vi "Update RPC Client Methods.vi"(7 "RPC Method Parameters":T1[](array[typedef]), 8 "error in (no error)":errorcluster, 11 "Server class in":refnum<vi>) -> (0 "error out":errorcluster, 3 "Server class out":refnum<vi>)   [LabVIEW 2019, in "gRPC Template Creation Utility.lvlib"]
uses:
  gRPC Template Creation Utility.lvlib
  TypeDefs/RPC Method Parameters.ctl
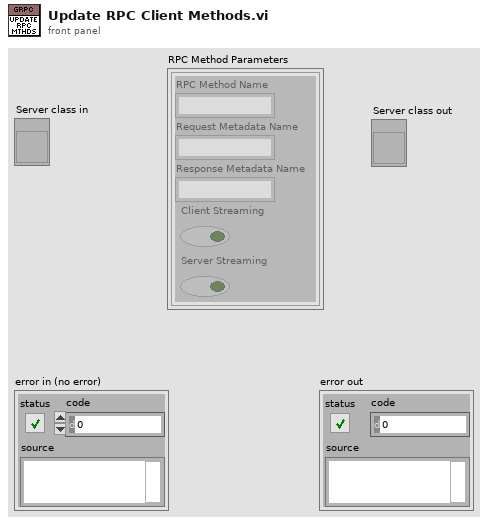
[diagram p1: front panel]
types:
  T1 = typedef "gRPC Template Creation Utility.lvlib/RPC Method Parameters.ctl" = cluster{"RPC Method Name":string, "Request Metadata Name":string, "Response Metadata Name":string, "Client Streaming":bool, "Server Streaming":bool}
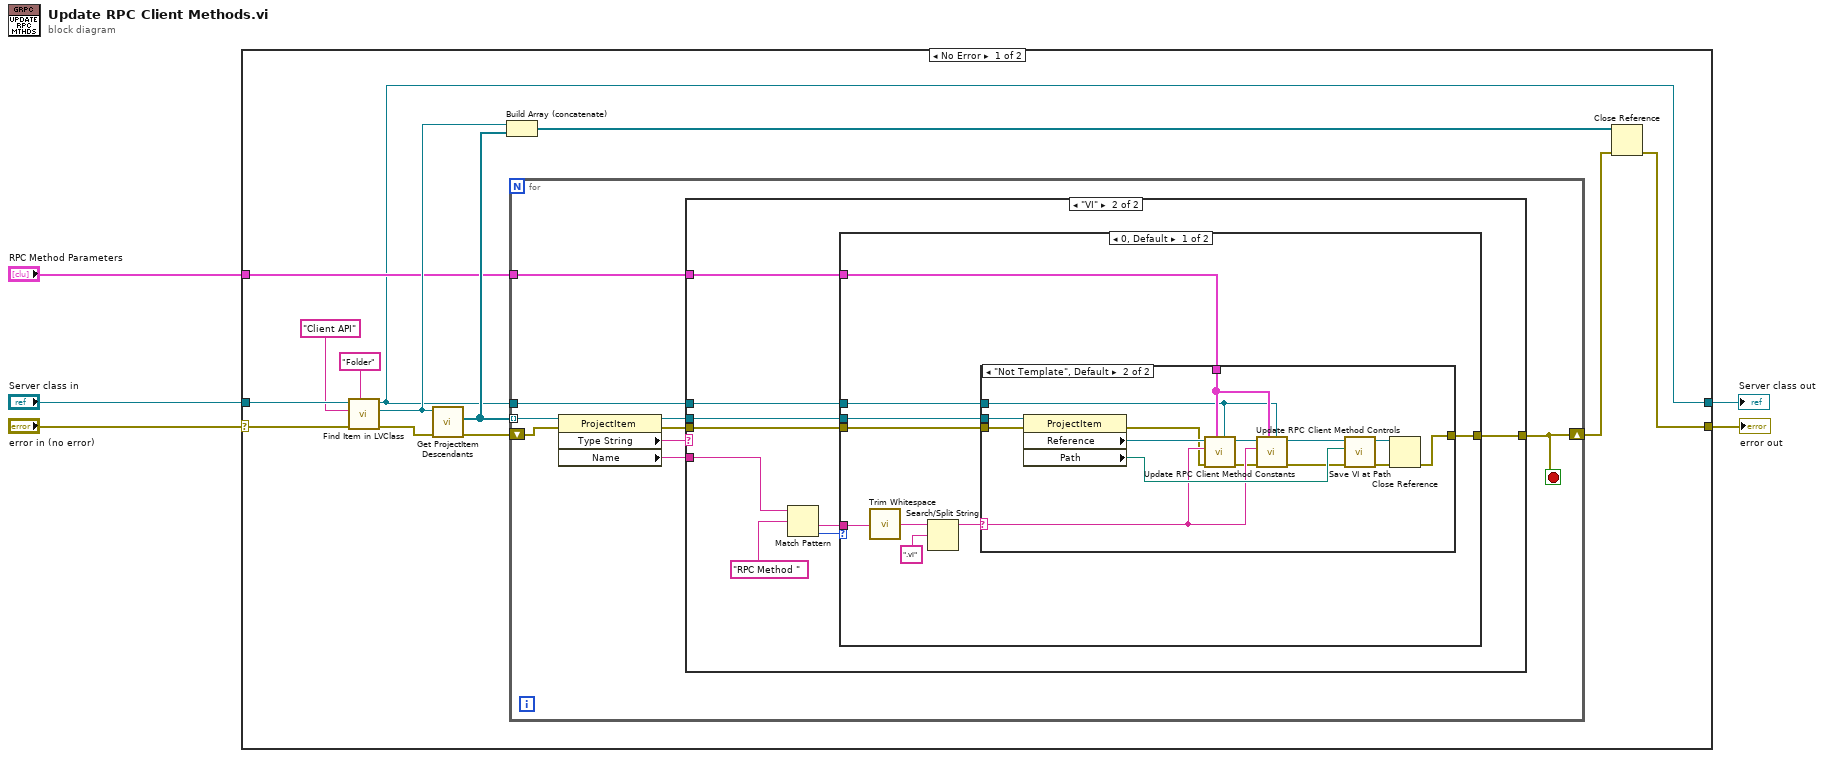
[diagram p0: block diagram]
diagram:
  n1 = case shown="No Error" "error in (no error)" {
    selector: "error in (no error)" -> [w9 w65]
    tunnel: [w7 w65] -> w5
    tunnel: "Server class in" -> [w13 w64]
    tunnel: "RPC Method Parameters" -> [w10 _]
    tunnel: [w6 w64] -> w1
    frame No Error {
      n2 = call "Find Item in LVClass.vi"("Item Type"="Folder", "error in (no error)"=w9, "Item Name"="Client API", "Class Item in"=w13) -> ("error out"=w14:errorcluster, "Project Item (Class Item)"=w15:refnum<vi>, "Class Item out"=w6:refnum<vi>)  [unwired: 4 in, 1 out]
      n3 = call "Get ProjectItem Descendants.vi"("error in (no error)"=w14, "ProjectItem in"=w15) -> ("error out"=w18:errorcluster, "All Descendents"=w16:refnum<vi>[])  [unwired: 7 in, 1 out]
      n4 = Build Array (concatenate)(w15, w16) -> (w17:refnum<vi>[])
      n5 = for {
        tunnel: w16 -> [w27] mode=indexing
        shift-right: [w21] -> w8
        shift-left: w18 -> [w24]
        tunnel: w10 -> [w20]
        tunnel: w6 -> [w19]
        stop <- w21 stop-if-true
        n6 = property class="ProjectItem"(reference=w27, error in=w24) -> (reference out=w25:refnum<vi>, error out=w23:errorcluster, "Type String"=w26:string, "Name"=w22:string)
        n7 = case shown="\"VI\"" w26 {
          tunnel: w25 -> [_ w35]
          tunnel: w23 -> [w28 w33]
          tunnel: w22 -> [_ w31]
          tunnel: [w28 w34] -> w21
          tunnel: w20 -> [_ w30]
          tunnel: w19 -> [_ w29]
          frame "None", Default {
          }
          frame "VI" {
            n8 = Match Pattern(string=w31, regular expression="RPC Method ") -> (after substring=w32:string, offset past match=w36:i32)  [unwired: 1 in, 2 out]
            n9 = case shown="0, Default" w36 {
              tunnel: w35 -> [w46 _]
              tunnel: [w43 w63] -> w34
              tunnel: w33 -> [w45 w63]
              tunnel: w32 -> [w42 _]
              tunnel: w30 -> [w44 _]
              tunnel: w29 -> [w38 _]
              frame 0, Default {
                n10 = call <vilib>:"Trim Whitespace.vi"("string"=w42) -> ("trimmed string"=w41:string)  [unwired: 1 in]
                n11 = Search/Split String(string=w41, search string/char (-)=".vi" ("regular expression")) -> (substring before match=w39:string)  [unwired: 1 in, 2 out]
                n12 = case shown="\"Not Template\", Default" w39 {
                  selector: w39 -> [_ w56]
                  tunnel: w46 -> [_ w62]
                  tunnel: w45 -> [w47 w61]
                  tunnel: w44 -> [_ w55]
                  tunnel: [w47 w60] -> w43
                  tunnel: w38 -> [_ w54]
                  frame "Template" {
                  }
                  frame "Not Template", Default {
                    n13 = property class="ProjectItem"(reference=w62, error in=w61) -> (error out=w52:errorcluster, "Reference"=w53:refnum<vi>, "Path"=w57:path)  [unwired: 1 out]
                    n14 = call "Update RPC Client Method Constants.vi"("Server class in"=w54, "RPC Method Parameters"=w55, "error in (no error)"=w52, "RPC Method Name"=w56, "VI in"=w53) -> ("error out"=w51:errorcluster, "VI out"=w48:refnum<vi>)  [unwired: 5 in]
                    n15 = call "Update RPC Client Method Controls.vi"("Server class in"=w54, "RPC Method Parameters"=w55, "error in (no error)"=w51, "RPC Method Name"=w56, "VI in"=w48) -> ("error out"=w50:errorcluster, "VI out"=w49:refnum<vi>)  [unwired: 5 in]
                    n16 = call "Save VI at Path.vi"("error in (no error)"=w50, "Path"=w57, "VI in"=w49) -> ("error out"=w59:errorcluster, "VI out"=w58:refnum<vi>)  [unwired: 6 in, 1 out]
                    n17 = Close Reference(reference=w58, error in (no error)=w59) -> (error out=w60:errorcluster)
                  }
                }
              }
              frame -1 {
              }
            }
          }
        }
      }
      n18 = Close Reference(reference=w17, error in (no error)=w8) -> (error out=w7:errorcluster)
    }
    frame Error {
    }
  }
  "error out" <- w5
  "Server class out" <- w1
